vi "serverState.vi"(7 "function":enum16{"set", "get"}(ring)=enum."get", 8 "error in (no error)":errorcluster, 10 "state":enum16{"stop", "run"}(ring)=enum."run") -> (0 "error out":errorcluster, 2 "state":enum16{"stop", "run"}(ring))   [LabVIEW 2018, in "TcpServer.lvclass"]
doc: "This is a FGV (must be replaced) that only informs to the Tcp Server was turned off and cheks the state of it."
uses:
  TcpServer.lvclass
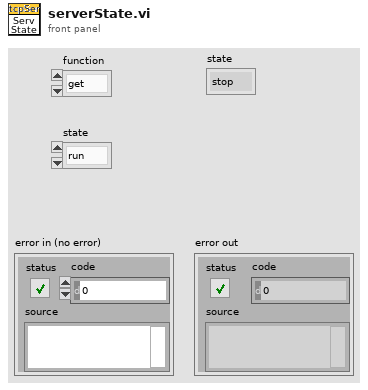
[diagram p1: front panel]
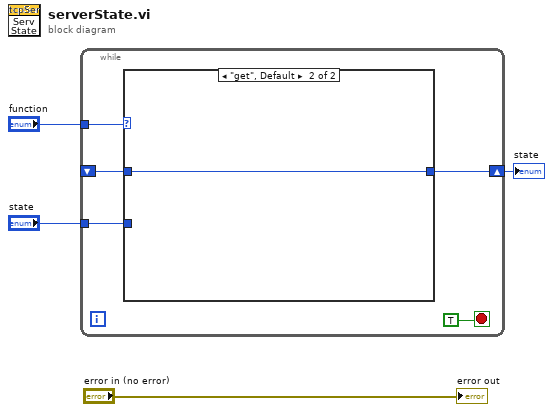
[diagram p0: block diagram]
diagram:
  n1 = while {
    tunnel: "function" -> [w8]
    tunnel: "state" -> [w7]
    shift-right: [w6] -> w1
    shift-left: _ -> [w5]
    stop <- TRUE stop-if-true
    n2 = case shown="\"get\", Default" w8 {
      tunnel: w7 -> [w10 _]
      tunnel: [w10 w11] -> w6
      tunnel: w5 -> [_ w11]
      frame "set" {
      }
      frame "get", Default {
      }
    }
  }
  "state" <- w1
  "error out" <- "error in (no error)"
